vi "Clip signal.vi"(4 "vel gain":dbl=0.1, 5 "max accel":dbl, 6 "pos gain":dbl=1.0, 7 "max speed":dbl, 8 "init vel":dbl, 9 "init pos":dbl, 10 "V":dbl[](array[numeric]), 11 "Y":dbl[](array[numeric])) -> (0 "final vel":dbl, 1 "final pos":dbl, 3 "Clipped Y":dbl[](array[numeric]))   [LabVIEW 2012]
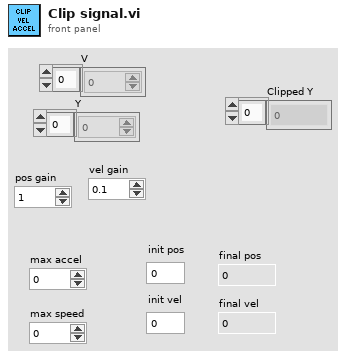
[diagram p1: front panel]
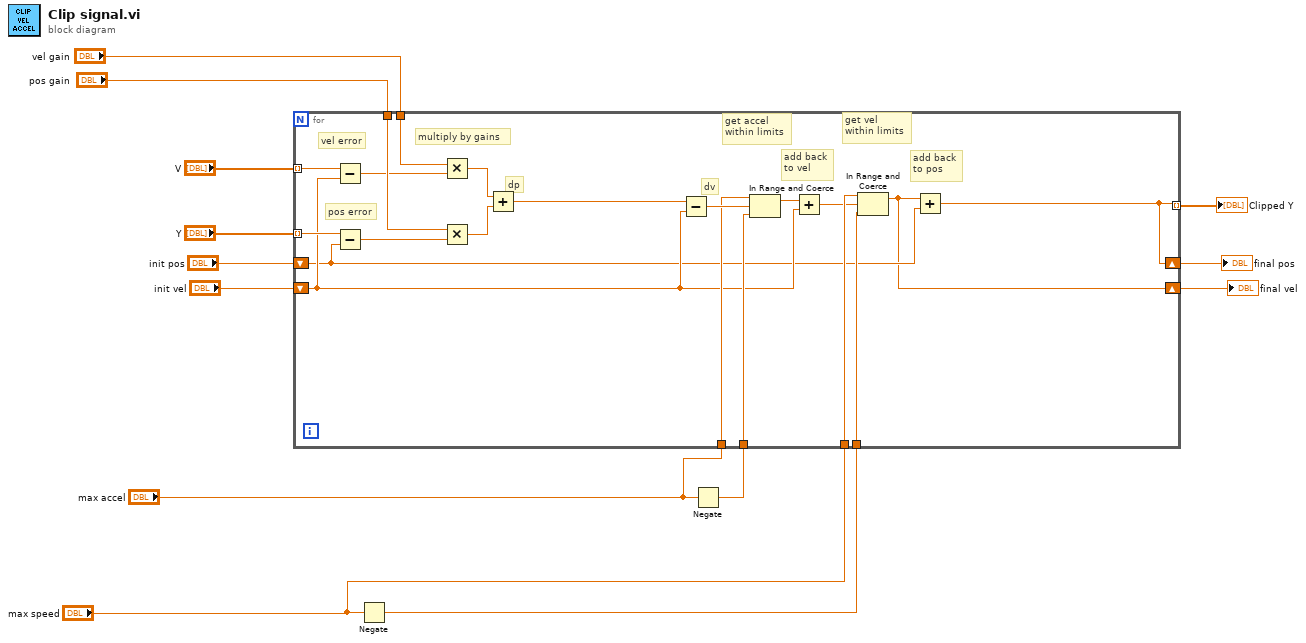
[diagram p0: block diagram]
diagram:
  n1 = Negate(x="max speed") -> (-x=w12:dbl)
  n2 = Negate(x="max accel") -> (-x=w13:dbl)
  n3 = for {
    tunnel: "Y" -> [w33] mode=indexing
    tunnel: "max accel" -> [w21]
    shift-right: [w15] -> w10
    shift-left: "init pos" -> [w17]
    shift-right: [w16] -> w9
    shift-left: "init vel" -> [w19]
    tunnel: w13 -> [w22]
    tunnel: w12 -> [w24]
    tunnel: "max speed" -> [w25]
    tunnel: "V" -> [w32] mode=indexing
    tunnel: "vel gain" -> [w31]
    tunnel: "pos gain" -> [w30]
    tunnel: [w15] -> w5 mode=indexing
    # "add back\nto pos"
    # "get vel\nwithin limits"
    # "add back\nto vel"
    # "get accel\nwithin limits"
    # "dv"
    # "dp"
    # "multiply by gains"
    # "pos error"
    # "vel error"
    n4 = Subtract(x=w32, y=w19) -> (x-y=w27:dbl)
    n5 = Subtract(x=w33, y=w17) -> (x-y=w26:dbl)
    n6 = Multiply(x=w31, y=w27) -> (x*y=w29:dbl)
    n7 = Multiply(x=w30, y=w26) -> (x*y=w28:dbl)
    n8 = Add(x=w29, y=w28) -> (x+y=w14:dbl)
    n9 = Subtract(x=w14, y=w19) -> (x-y=w23:dbl)
    n10 = In Range and Coerce(upper limit=w21, x=w23, lower limit=w22) -> (coerced(x)=w20:dbl)  [unwired: 1 out]
    n11 = Add(x=w20, y=w19) -> (x+y=w18:dbl)
    n12 = In Range and Coerce(upper limit=w25, x=w18, lower limit=w24) -> (coerced(x)=w16:dbl)  [unwired: 1 out]
    n13 = Add(x=w16, y=w17) -> (x+y=w15:dbl)
  }
  "final pos" <- w10
  "final vel" <- w9
  "Clipped Y" <- w5
